vi "Byte to Pixel Stream.vi"(1 "RGB Byte Stream":u8[](array[numeric]) format="0x%02x") -> (0 "Pixel Stream":u32[](array[numeric]) format="0x%08x")   [LabVIEW 2013]
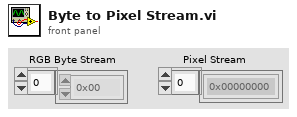
[diagram p1: front panel]
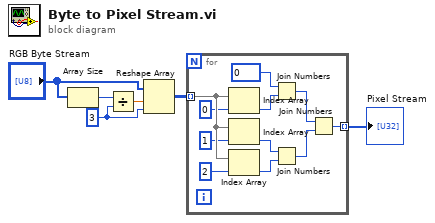
[diagram p0: block diagram]
diagram:
  w4 = 3
  n1 = Array Size(array="RGB Byte Stream") -> (size(s)=w5:i32)
  n2 = Divide(x=w5, y=w4) -> (x/y=w3:dbl)
  n3 = Reshape Array("RGB Byte Stream", w3, w4) -> (w2:u8[][])
  n4 = for {
    tunnel: w2 -> [w17] mode=indexing
    tunnel: [w7] -> w1 mode=indexing
    n5 = Index Array(array=w17, index=0) -> (element=w11:u8)
    n6 = Index Array(array=w17, index=1) -> (element=w13:u8)
    n7 = Index Array(array=w17, index=2) -> (element=w12:u8)
    n8 = Join Numbers(hi=u8 0, lo=w11) -> ((hi.lo)=w9:u16)
    n9 = Join Numbers(hi=w13, lo=w12) -> ((hi.lo)=w8:u16)
    n10 = Join Numbers(hi=w9, lo=w8) -> ((hi.lo)=w7:u32)
  }
  "Pixel Stream" <- w1
